vi "MeasurementServer_DetermineLibrary.vi"() -> (3 "path out":path)   [LabVIEW 2019, in "labview-grpc-measurement-server.lvlib"]
uses:
  labview-grpc-measurement-server.lvlib
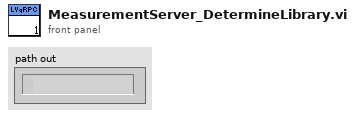
[diagram p1: front panel]
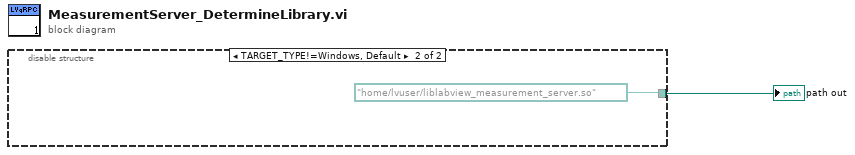
[diagram p0: block diagram]
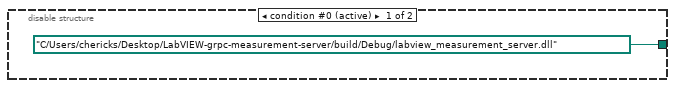
[diagram p2: hidden frame]
diagram:
  n1 = disable-structure shown="TARGET_TYPE!=Windows, Default" {
    disable-tunnel: [path "C:/Users/chericks/Desktop/LabVIEW-grpc-measurement-server/build/Debug/labview_measurement_server.dll" ("path in") path "/home/lvuser/liblabview_measurement_server.so" ("path in")] -> w1
    frame condition #0 (active) {
    }
    frame condition #1 {
    }
  }
  "path out" <- w1
